vi "Priority.vi"(8 "error in (no error)":errorcluster, 11 "Authentication Handler in":refnum<class "Authentication Handler.lvclass">) -> (0 "error out":errorcluster, 2 "Priority":u16, 3 "Authentication Handler out":refnum<class "Authentication Handler.lvclass">)   [LabVIEW 2020, in "HTTP Server.lvlib" / "Authentication Handler.lvclass"]
uses:
  Authentication Handler.lvclass
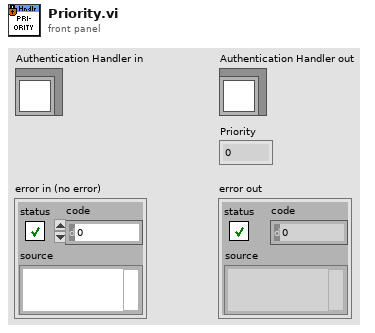
[diagram p1: front panel]
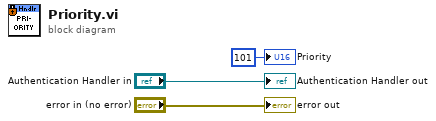
[diagram p0: block diagram]
diagram:
  "error out" <- "error in (no error)"
  "Authentication Handler out" <- "Authentication Handler in"
  "Priority" <- u16 101 ("Priority")
